vi "Auto Generator.vi"() -> ()   [LabVIEW 2014]
uses:
  <vilib>/FTP/NI_FTP.lvlib
panel:
  in  "Instructions":T1(array[cluster])
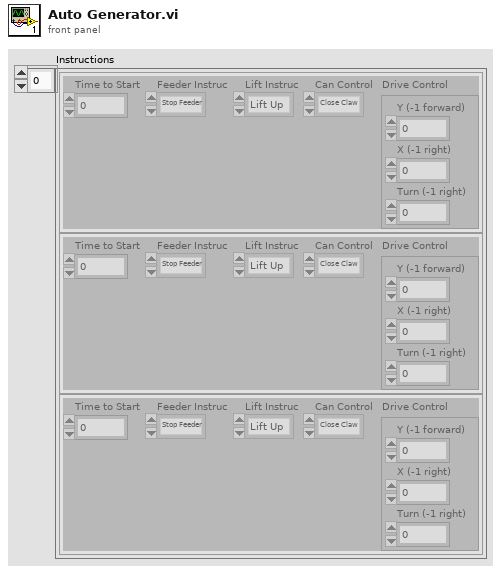
[diagram p1: front panel]
types:
  T1 = cluster{"Time to Start":dbl, "Feeder Instruc":enum16{"Stop Feeder", "Infeed", "Outfeed", "Rightfeed", "Leftfeed"}, "Lift Instruc":enum16{"Lift Up", "Lift Down"}, "Can Control":enum16{"Close Claw", "Open Claw", "Fast Up", "Slow Up", "Stop", "Srow Down", "Fast Down"}, "Drive Control":cluster{"Y (-1 forward) ":dbl, "X (-1 right)":dbl, "Turn (-1 right)":dbl}}[]
  T2 = enum16{"open", "replace", "create", "open or create", "replace or create", "replace or create with confirmation"}
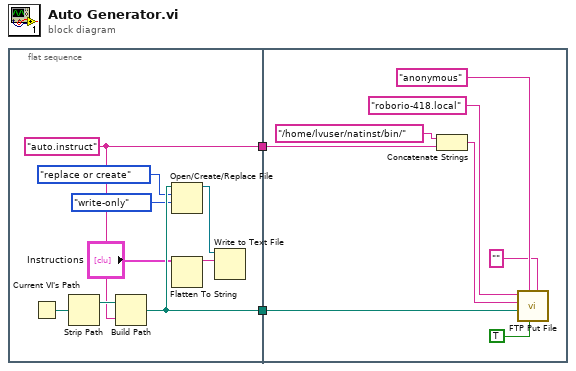
[diagram p0: block diagram]
diagram:
  n1 = flat-sequence {
    tunnel: [w9] -> w2
    tunnel: [w4] -> w1
    tunnel: w2 -> [w16]
    tunnel: w1 -> [w14]
    frame #0 {
      w4 = "auto.instruct" ("name or relative path")
      n2 = Current VI's Path() -> (path=w5:path)
      n3 = Strip Path(path=w5) -> (stripped path=w6:path)  [unwired: 1 out]
      n4 = Build Path(base path=w6, name or relative path=w4) -> (appended path=w9:path)
      n5 = Open/Create/Replace File(file path (use dialog)=w9, operation (0:open)=T2."replace or create", access (0:read/write)=enum16{"read/write", "read-only", "write-only"}."write-only") -> (refnum out=w10:refnum<file>)  [unwired: 3 in, 2 out]
      n6 = Flatten To String(anything="Instructions") -> (data string=w11:string)  [unwired: 3 in, 2 out]
      n7 = Write to Text File(file (use dialog)=w10, text=w11) -> ()  [unwired: 2 in, 3 out]
    }
    frame #1 {
      n8 = Concatenate Strings("/home/lvuser/natinst/bin/" ("remote path"), w14) -> (w13:string)
      n9 = call <vilib>:"FTP Put File.vi"("password"="", "binary (F)"=TRUE, "user"="anonymous", "local path"=w16, "remote path"=w13, "host"="roborio-418.local") -> ()  [unwired: 4 in, 2 out]
    }
  }
